vi "Get Request Type.vi"(8 "error in (no error)":errorcluster, 11 "GetSceneCollectionList in":refnum<class "GetSceneCollectionList.lvclass">) -> (0 "error out":errorcluster, 2 "Request Type":string, 3 "GetSceneCollectionList out":refnum<class "GetSceneCollectionList.lvclass">)   [LabVIEW 2020, in "obs-websocket.lvlib" / "GetSceneCollectionList.lvclass"]
uses:
  GetSceneCollectionList.lvclass
  GetSceneCollectionList.lvclass/GetSceneCollectionList.ctl
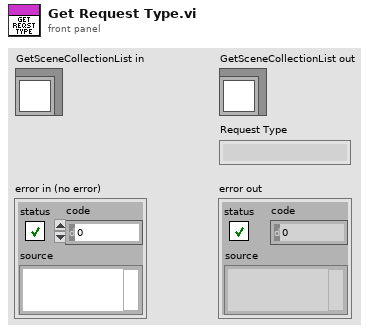
[diagram p1: front panel]
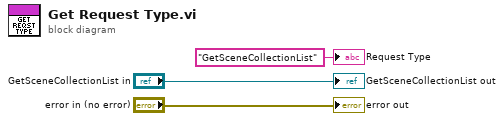
[diagram p0: block diagram]
diagram:
  "error out" <- "error in (no error)"
  "GetSceneCollectionList out" <- "GetSceneCollectionList in"
  "Request Type" <- "GetSceneCollectionList" ("Request Type")
